vi "Teardown.vi"(7 "Sender":refnum<class "Sender.lvclass">, 11 "TEMPLATE jettl in":refnum<class "TEMPLATE jettl.lvclass">) -> (3 "TEMPLATE jettl out":refnum<class "TEMPLATE jettl.lvclass">)   [LabVIEW 2021, in "_Template.lvlib" / "Templates.lvlib" / "TEMPLATE jettl.lvlib" / "TEMPLATE jettl.lvclass"]
uses:
  TEMPLATE jettl.lvclass
  TEMPLATE jettl.lvclass/TEMPLATE jettl.ctl
  jettl/jettl/jettl/jettl.lvclass
  jettl/jettl/Sender/Sender/Sender.lvclass
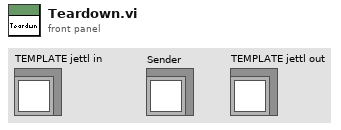
[diagram p1: front panel]
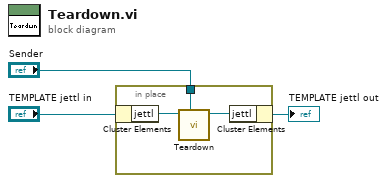
[diagram p0: block diagram]
diagram:
  n1 = in-place {
    in-place-border: "Sender" -> [w4]
    n2 = in-place-cluster #1("TEMPLATE jettl in") -> ("jettl"=w6:refnum<class "jettl.lvclass">)
    n3 = call-dynamic "Teardown.vi"("Sender"=w4, "Teardown in"=w6) -> ("Teardown out"=w5:refnum<class "jettl.lvclass">)  [unwired: 9 in]
    n4 = in-place-cluster #1("jettl"=w5) -> (→"TEMPLATE jettl out":refnum<class "TEMPLATE jettl.lvclass">)
  }
